vi "Setup manipulator (SubVI).vi"(1 "G_upper bound":i32, 3 "M_lower bound":i32, 11 "error in (no error)":errorcluster, 12 "M_Encoder Ref In":T1, 14 "G_Encoder Ref In":T1) -> (15 "error out":errorcluster)   [LabVIEW 2017]
uses:
  <vilib>/myRIO/Instrument Drivers/Onboard IO/Encoder/typedefs/Encoder Reference.ctl
  <vilib>/myRIO/Common/Instrument Driver Framework/Utilities/typedefs/myRIO Generic Hardware Reference.ctl
  <vilib>/myRIO/Common/Instrument Driver Framework/Utilities/typedefs/Hardware Version Enum.ctl
  <vilib>/myRIO/Common/Instrument Driver Framework/Utilities/typedefs/myRIO v1.0 Reference.ctl
  <vilib>/myRIO/Common/Instrument Driver Framework/Utilities/typedefs/Generic FPGA Reference.ctl
  <vilib>/myRIO/Common/Instrument Driver Framework/myRIO v1.0/Encoder/typedefs/Encoder Channels Enum.ctl
  <vilib>/myRIO/Instrument Drivers/Onboard IO/DIO/typedefs/DIO Reference.ctl
  <vilib>/myRIO/Common/Instrument Driver Framework/myRIO v1.0/DIO/typedefs/DIO Channels List.ctl
  <vilib>/myRIO/Common/Instrument Driver Framework/myRIO v1.0/DIO/typedefs/DIO Channels Enum.ctl
  <vilib>/userdefined/High Color/nirio_resource_hc.ctl
  <vilib>/myRIO/Common/Instrument Driver Framework/Utilities/vis/Is FPGA Ref Available.vi
  <vilib>/myRIO/Common/Instrument Driver Framework/myRIO v1.0/DIO/vis/myRIO v1.1 Open DIO.vi
  <vilib>/myRIO/Instrument Drivers/Onboard IO/DIO/vis/Write.vi
  <vilib>/myRIO/Common/Instrument Driver Framework/Utilities/vis/Validate Channels.vi
  <vilib>/myRIO/Common/Instrument Driver Framework/myRIO v1.0/DIO/vis/myRIO v1.0 Reserve DIO.vi
  <vilib>/myRIO/Common/Instrument Driver Framework/myRIO v1.0/Resource Manager/vis/myRIO v1.0 Reserve Channel List.vi
  <vilib>/myRIO/Common/Instrument Driver Framework/myRIO v1.0/DIO/vis/myRIO v1.0 Build MUX Configuration DIO.vi
  <vilib>/myRIO/Common/Instrument Driver Framework/myRIO v1.0/Resource Manager/vis/myRIO v1.0 Reserve Channel.vi
  <vilib>/myRIO/Common/Instrument Driver Framework/myRIO v1.0/Resource Manager/vis/myRIO v1.0 Unreserve Channel.vi
  <vilib>/myRIO/Common/Instrument Driver Framework/myRIO v1.0/Resource Manager/vis/myRIO v1.0 Create Configuration List.vi
  <vilib>/myRIO/Common/Instrument Driver Framework/myRIO v1.0/Resource Manager/vis/myRIO v1.0 Build Mutex Name.vi
  <vilib>/Utility/error.llb/Error Cluster From Error Code.vi
  <vilib>/myRIO/Common/Instrument Driver Framework/myRIO v1.0/Encoder/vis/myRIO v1.0 Read Encoder.vi
  <vilib>/Utility/VariantDataType/GetNumericInfo.vi
  <vilib>/myRIO/Common/Instrument Driver Framework/myRIO v1.0/myRIO v1.1 Open.vi
  <vilib>/myRIO/Common/Instrument Driver Framework/Utilities/vis/IO Manager.vi
  <vilib>/myRIO/Common/Instrument Driver Framework/Utilities/vis/Configuration Manager.vi
  <vilib>/myRIO/Common/Instrument Driver Framework/myRIO v1.0/Resource Manager/vis/myRIO v1.0 Configure IO.vi
  <vilib>/myRIO/Common/Instrument Driver Framework/myRIO v1.0/myRIO v1.0 Close.vi
  <vilib>/myRIO/Common/Instrument Driver Framework/myRIO v1.0/DIO/vis/myRIO v1.0 Write DIO.vi
  <vilib>/myRIO/Express VI/Onboard IO/DO/DO Express VI.xnode
  <vilib>/myRIO/Instrument Drivers/Onboard IO/DIO/vis/myRIO DIO Open.xnode
  <vilib>/myRIO/Instrument Drivers/Onboard IO/Encoder/Encoder.lvlib
  <vilib>/myRIO/Instrument Drivers/Onboard IO/DIO/DIO.lvlib
panel:
  out "reversedG":bool
  out "reversedM":bool
  in  "offset for Extra Stop":i32=100
  in  "iterations control":i32=10
  in  "offset":i32=50
  in  "frames to pass":i32=100
  in  "def it":i32=100
  out "ArrG_enc_val":i32[](array[numeric])
  out "ArrM_enc_val":i32[](array[numeric])
  in  "G+ (B/DIO13 (Pin 26))":bool
  in  "G- (B/DIO7 (Pin 25))":bool
  in  "M- (B/DIO6 (Pin 23))":bool
  in  "M+ (B/DIO5 (Pin 21))":bool
  in  "stopG":bool
  out "G+":bool
  out "G enc val":i32
  out "M+":bool
  in  "stopM":bool
  out "M enc val":i32
  # "EXTRA STOP CONTROLS"
  # "SET UP THE VALUES"
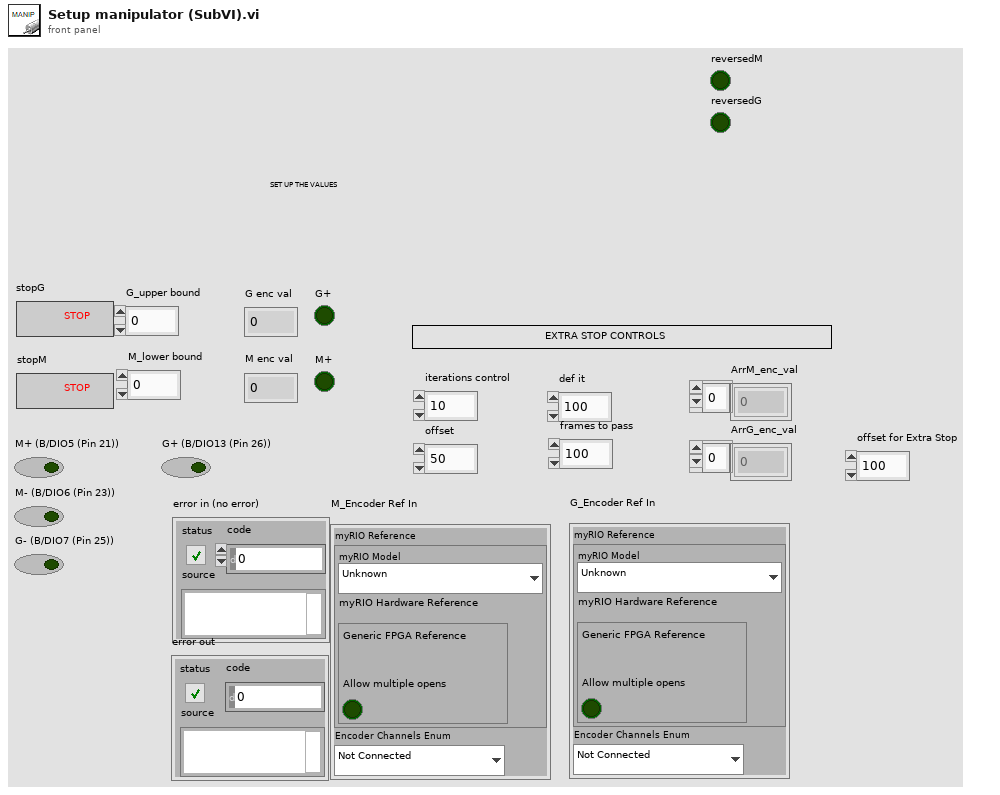
[diagram p1: front panel]
types:
  T1 = typedef "Encoder.lvlib/Encoder Reference.ctl" = cluster{"myRIO Reference":T2, "Encoder Channels Enum":T6}
  T2 = typedef "myRIO Generic Hardware Reference.ctl" = cluster{"myRIO Model":T3, "myRIO Hardware Reference":T4}
  T3 = typedef "Hardware Version Enum.ctl" = enum16{"Unknown", "myRIO-1900", "myRIO-1950", "roboRIO", "NI ELVIS RIO CM"}
  T4 = typedef "myRIO v1.0 Reference.ctl" = cluster{"Generic FPGA Reference":T5, "Allow multiple opens":bool}
  T5 = typedef "Generic FPGA Reference.ctl" = refnum<k20>
  T6 = typedef "Encoder Channels Enum.ctl" = enum16{"Not Connected", "C/ENC0", "C/ENC1", "A/ENC", "B/ENC", "DIO/ENC0", "DIO/ENC1", "DIO/ENC2", "DIO/ENC3", "DIO/ENC4"}
  T7 = typedef "DIO.lvlib/DIO Reference.ctl" = cluster{"myRIO Reference":T2, "DIO Channels List":T8}
  T8 = typedef "DIO Channels List.ctl" = T9[]
  T9 = typedef "DIO Channels Enum.ctl" = enum16{"Not Connected", "C/DIO0", "C/DIO1", "C/DIO2", "C/DIO3", "C/DIO4", "C/DIO5", "C/DIO6", "C/DIO7", "A/DIO0", "A/DIO1", "A/DIO2", "A/DIO3", "A/DIO4", "A/DIO5", "A/DIO6", "A/DIO7", "A/DIO8", "A/DIO9", "A/DIO10", "A/DIO11", "A/DIO12", "A/DIO13", "A/DIO14", "A/DIO15", "B/DIO0", "B/DIO1", "B/DIO2", "B/DIO3", "B/DIO4", "B/DIO5", "B/DIO6", "B/DIO7", "B/DIO8", "B/DIO9", "B/DIO10", "B/DIO11", "B/DIO12", "B/DIO13", "B/DIO14", "B/DIO15", "LED0", "LED1", "LED2", "LED3", "Button0", "DIO/DIO0", "DIO/DIO1", "DIO/DIO2", "DIO/DIO3", "DIO/DIO4", "DIO/DIO5", "DIO/DIO6", "DIO/DIO7", "DIO/DIO8", "DIO/DIO9", "SPI/CS0", "SPI/CS1", "SPI/CS2", "SPI/CS3", "LED RADIO (Green)", "LED RADIO (Red)", "LED COMM (Green)", "LED COMM (Red)", "LED MODE (Green)", "LED MODE (Red)"}
  T10 = typedef "nirio_resource_hc.ctl" = tag
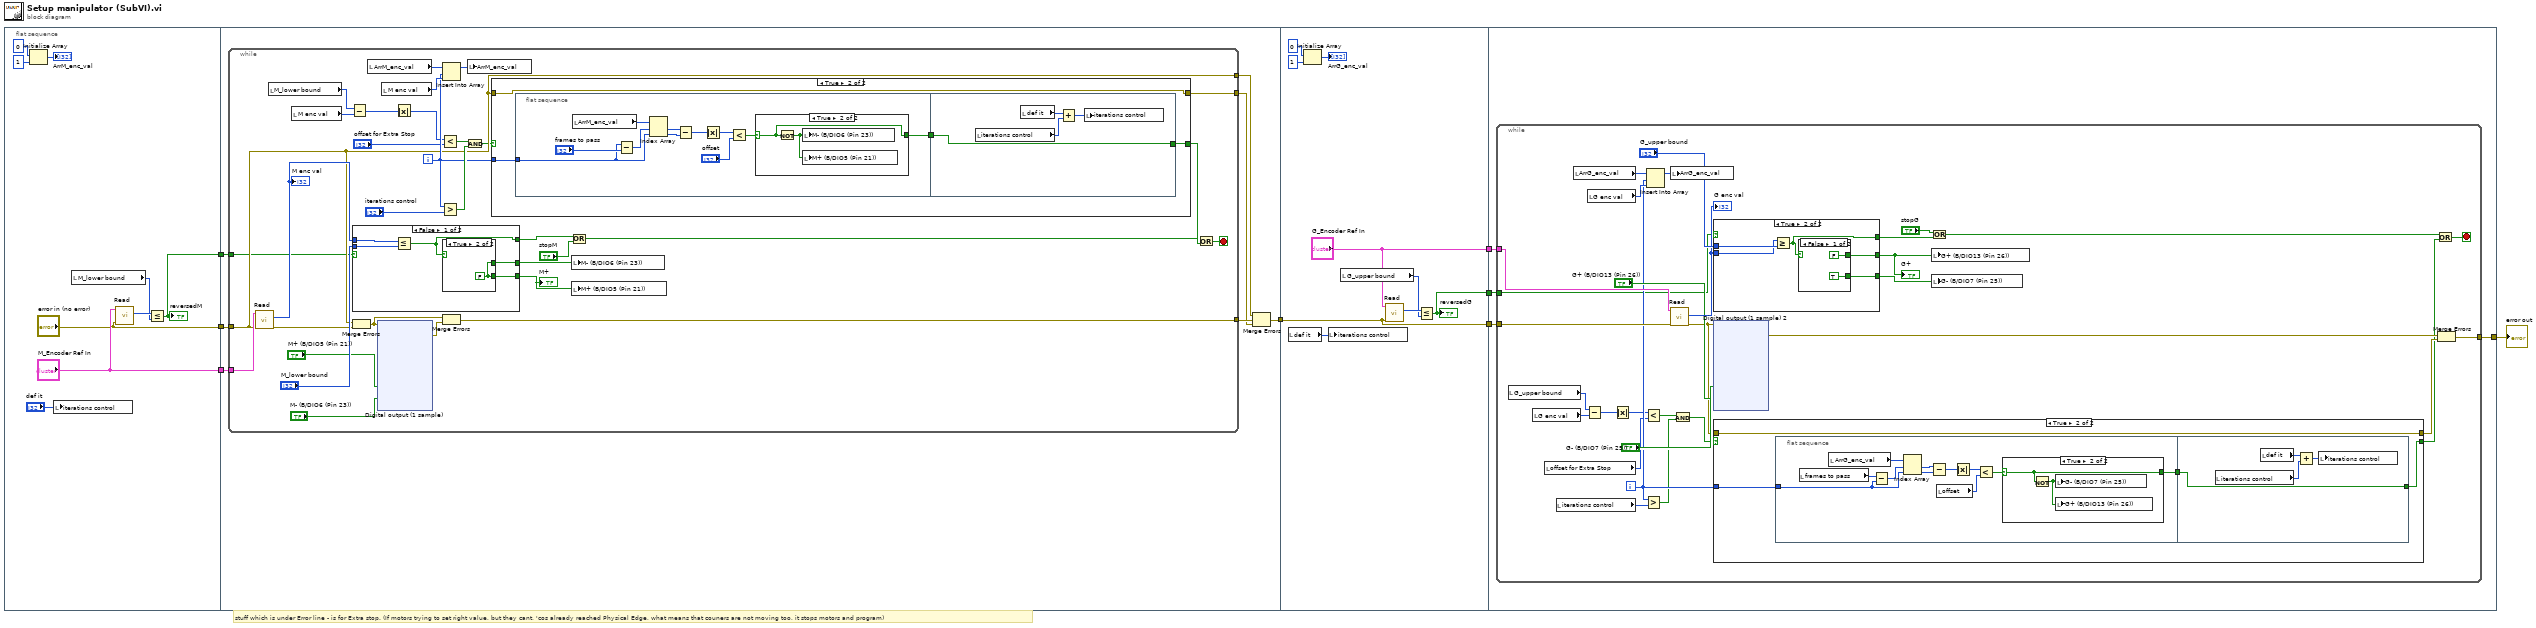
[diagram p0: block diagram]
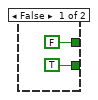
[diagram p4: hidden frame]
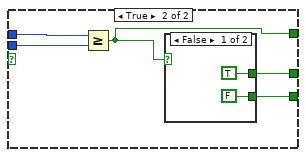
[diagram p5: hidden frame]
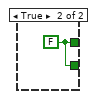
[diagram p6: hidden frame]
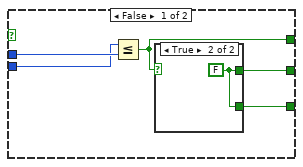
[diagram p9: hidden frame]
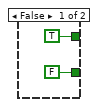
[diagram p10: hidden frame]
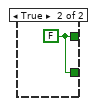
[diagram p11: hidden frame]
diagram:
  # "stuff which is under Error line - is for Extra stop. (If motors trying to set right value, but they cant, 'cos already reached Physical Edge, what means that couners are not moving too, it stops motors and program)"
  n1 = flat-sequence {
    tunnel: ["error in (no error)"] -> w8
    tunnel: ["M_Encoder Ref In"] -> w7
    tunnel: [w9] -> w1
    tunnel: w8 -> [w24]
    tunnel: w7 -> [w21]
    tunnel: [w20] -> w6
    tunnel: w1 -> [w18]
    tunnel: w6 -> [w136]
    tunnel: [w136] -> w5
    tunnel: ["G_Encoder Ref In"] -> w4
    tunnel: [w133] -> w2
    tunnel: w5 -> [w145]
    tunnel: w4 -> [w144]
    tunnel: [w143] -> w3
    tunnel: w2 -> [w142]
    frame #0 {
      n2 = Initialize Array(0 ("dimension size"), 1 ("dimension size")) -> (→"ArrM_enc_val":i32[])
      n3 = local write "iterations control"("def it") -> ()
      n4 = local read "M_lower bound"() -> (w10:i32)
      n5 = call <vilib>:"Read.vi"("error in (no error)"="error in (no error)", "Encoder Ref In"="M_Encoder Ref In") -> ("Counter Value"=w11:i32)  [unwired: 5 in, 4 out]
      n6 = Less Or Equal?(x=w11, y=w10) -> (x <= y?=w9:bool)
      "reversedM" <- w9
    }
    frame #1 {
      n7 = while {
        tunnel: w24 -> [w40]
        tunnel: [w40] -> w23
        tunnel: [w55] -> w22
        tunnel: w21 -> [w54]
        tunnel: [w39] -> w19
        tunnel: w18 -> [w25]
        i -> [w41]
        stop <- w37 stop-if-true
        n8 = call <vilib>:"Read.vi"("error in (no error)"=w40, "Encoder Ref In"=w54) -> ("error out"=w53:errorcluster, "Counter Value"=w52:i32)  [unwired: 5 in, 3 out]
        "M enc val" <- w52
        n9 = local read "M_lower bound"() -> (w30:i32)
        n10 = local read "M enc val"() -> (w31:i32)
        n11 = Subtract(x=w30, y=w31) -> (x-y=w28:i32)
        n12 = case shown="False" w25 {
          tunnel: "M_lower bound" -> [w85 w93]
          tunnel: [w81 w89] -> w48
          tunnel: w52 -> [w84 w92]
          tunnel: [w83 w90] -> w34
          tunnel: [w82 w91] -> w33
          frame False {
            n13 = Less Or Equal?(x=w84, y=w85) -> (x <= y?=w81:bool)
            n14 = case shown="True" w81 {
              tunnel: [TRUE w88] -> w83
              tunnel: [FALSE w88] -> w82
              frame False {
              }
              frame True {
                w88 = FALSE
              }
            }
          }
          frame True {
            n15 = Greater Or Equal?(x=w92, y=w93) -> (x >= y?=w89:bool)
            n16 = case shown="False" w89 {
              tunnel: [TRUE ("M- (B/DIO6 (Pin 23))") w96] -> w91
              tunnel: [FALSE ("M- (B/DIO6 (Pin 23))") w96] -> w90
              frame False {
              }
              frame True {
                w96 = FALSE
              }
            }
          }
        }
        "M+" <- w34
        n17 = Merge Errors(w40, w53) -> (w49:errorcluster)
        n18 = local read "ArrM_enc_val"() -> (w44:i32[])
        n19 = xnode "Digital output (1 sample)"("M+ (B/DIO5 (Pin 21))"="M+ (B/DIO5 (Pin 21))", "M- (B/DIO6 (Pin 23))"="M- (B/DIO6 (Pin 23))", "error in (no error)"=w49) -> ("error out"=w50:errorcluster)
        n20 = local read "M enc val"() -> (w42:i32)
        n21 = Absolute Value(x=w28) -> (abs(x)=w26:i32)
        n22 = Less?(x=w26, y="offset for Extra Stop") -> (x < y?=w29:bool)
        n23 = Greater?(x=w41, y="iterations control") -> (0:w46:bool)
        n24 = Insert Into Array(array=w44, index=w41, new element=w42) -> (w43:i32[])
        n25 = Merge Errors(w49, w50) -> (w55:errorcluster)
        n26 = And(x=w29, y=w46) -> (x .and. y?=w32:bool)
        n27 = local write "ArrM_enc_val"(w43) -> ()
        n28 = case shown="True" w32 {
          selector: w32 -> [w57 _]
          tunnel: w41 -> [_ w62]
          tunnel: w40 -> [w58 w61]
          tunnel: [w58 w61] -> w39
          tunnel: [w57 w59] -> w47
          frame False {
          }
          frame True {
            n29 = flat-sequence {
              tunnel: w62 -> [w70]
              tunnel: [w63] -> w60
              tunnel: [w77] -> w59
              tunnel: w60 -> [w77]
              frame #0 {
                n30 = local read "ArrM_enc_val"() -> (w73:i32[])
                n31 = Subtract(x=w70, y="frames to pass") -> (x-y=w71:i32)
                n32 = Index Array(array=w73, index #1=w71, index #2=w70) -> (element #1=w69:i32, element #2=w68:i32)
                n33 = Subtract(x=w69, y=w68) -> (x-y=w67:i32)
                n34 = Absolute Value(x=w67) -> (abs(x)=w66:i32)
                n35 = Less?(x=w66, y="offset") -> (x < y?=w64:bool)
                n36 = case shown="True" w64 {
                  selector: w64 -> [w74 w75]
                  tunnel: [w74 w75] -> w63
                  frame False {
                  }
                  frame True {
                    n37 = Not(x=w75) -> (.not. x?=w76:bool)
                    n38 = local write "M- (B/DIO6 (Pin 23))"(w76) -> ()
                    n39 = local write "M+ (B/DIO5 (Pin 21))"(w76) -> ()
                  }
                }
              }
              frame #1 {
                n40 = local read "iterations control"() -> (w80:i32)
                n41 = local read "def it"() -> (w78:i32)
                n42 = Add(x=w78, y=w80) -> (x+y=w79:i32)
                n43 = local write "iterations control"(w79) -> ()
              }
            }
          }
        }
        n44 = Or(x=w48, y="stopM") -> (x .or. y?=w38:bool)
        n45 = local write "M- (B/DIO6 (Pin 23))"(w33) -> ()
        n46 = local write "M+ (B/DIO5 (Pin 21))"(w34) -> ()
        n47 = Or(x=w38, y=w47) -> (x .or. y?=w37:bool)
      }
      n48 = Merge Errors(w23, w22, w19) -> (w20:errorcluster)
    }
    frame #2 {
      n49 = local read "def it"() -> (w139:i32)
      n50 = Initialize Array(0 ("dimension size"), 1 ("dimension size")) -> (→"ArrG_enc_val":i32[])
      n51 = local write "iterations control"(w139) -> ()
      n52 = local read "G_upper bound"() -> (w134:i32)
      n53 = call <vilib>:"Read.vi"("error in (no error)"=w136, "Encoder Ref In"="G_Encoder Ref In") -> ("Counter Value"=w135:i32)  [unwired: 5 in, 4 out]
      n54 = Less Or Equal?(x=w135, y=w134) -> (x <= y?=w133:bool)
      "reversedG" <- w133
    }
    frame #3 {
      n55 = while {
        tunnel: w145 -> [w174]
        tunnel: [w159] -> w143
        tunnel: w144 -> [w170]
        tunnel: w142 -> [w146]
        i -> [w161]
        stop <- w156 stop-if-true
        n56 = local read "G_upper bound"() -> (w150:i32)
        n57 = local read "G enc val"() -> (w151:i32)
        n58 = local read "offset for Extra Stop"() -> (w149:i32)
        n59 = local read "iterations control"() -> (w163:i32)
        n60 = local read "ArrG_enc_val"() -> (w164:i32[])
        n61 = Subtract(x=w150, y=w151) -> (x-y=w152:i32)
        n62 = local read "G enc val"() -> (w165:i32)
        n63 = Absolute Value(x=w152) -> (abs(x)=w147:i32)
        n64 = Less?(x=w147, y=w149) -> (x < y?=w148:bool)
        n65 = Greater?(x=w161, y=w163) -> (0:w157:bool)
        n66 = Insert Into Array(array=w164, index=w161, new element=w165) -> (w162:i32[])
        n67 = local write "ArrG_enc_val"(w162) -> ()
        n68 = call <vilib>:"Read.vi"("error in (no error)"=w174, "Encoder Ref In"=w170) -> ("error out"=w160:errorcluster, "Counter Value"=w175:i32)  [unwired: 5 in, 3 out]
        "G enc val" <- w175
        n69 = And(x=w148, y=w157) -> (x .and. y?=w153:bool)
        n70 = case shown="True" w146 {
          tunnel: "G_upper bound" -> [w205 w213]
          tunnel: w175 -> [w204 w212]
          tunnel: [w201 w209] -> w172
          tunnel: [w203 w210] -> w167
          tunnel: [w202 w211] -> w166
          frame False {
            n71 = Less Or Equal?(x=w204, y=w205) -> (x <= y?=w201:bool)
            n72 = case shown="True" w201 {
              tunnel: [TRUE w208] -> w203
              tunnel: [FALSE w208] -> w202
              frame False {
              }
              frame True {
                w208 = FALSE
              }
            }
          }
          frame True {
            n73 = Greater Or Equal?(x=w212, y=w213) -> (x >= y?=w209:bool)
            n74 = case shown="False" w209 {
              tunnel: [TRUE w216] -> w211
              tunnel: [FALSE w216] -> w210
              frame False {
              }
              frame True {
                w216 = FALSE
              }
            }
          }
        }
        "G+" <- w167
        n75 = xnode "Digital output (1 sample) 2"("G- (B/DIO7 (Pin 25))"="G- (B/DIO7 (Pin 25))", "G+ (B/DIO13 (Pin 26))"="G+ (B/DIO13 (Pin 26))", "error in (no error)"=w160) -> ("error out"=w171:errorcluster)
        n76 = case shown="True" w153 {
          selector: w153 -> [w177 _]
          tunnel: w161 -> [_ w182]
          tunnel: w160 -> [w178 w181]
          tunnel: [w178 w181] -> w158
          tunnel: [w177 w180] -> w154
          frame False {
          }
          frame True {
            n77 = flat-sequence {
              tunnel: w182 -> [w188]
              tunnel: [w183] -> w179
              tunnel: [w197] -> w180
              tunnel: w179 -> [w197]
              frame #0 {
                n78 = local read "frames to pass"() -> (w186:i32)
                n79 = local read "ArrG_enc_val"() -> (w193:i32[])
                n80 = Subtract(x=w186, y=w188) -> (x-y=w187:i32)
                n81 = Index Array(array=w193, index #1=w187, index #2=w188) -> (element #1=w190:i32, element #2=w185:i32)
                n82 = Subtract(x=w190, y=w185) -> (x-y=w192:i32)
                n83 = local read "offset"() -> (w184:i32)
                n84 = Absolute Value(x=w192) -> (abs(x)=w191:i32)
                n85 = Less?(x=w191, y=w184) -> (x < y?=w189:bool)
                n86 = case shown="True" w189 {
                  selector: w189 -> [w194 w195]
                  tunnel: [w194 w195] -> w183
                  frame False {
                  }
                  frame True {
                    n87 = Not(x=w195) -> (.not. x?=w196:bool)
                    n88 = local write "G- (B/DIO7 (Pin 25))"(w196) -> ()
                    n89 = local write "G+ (B/DIO13 (Pin 26))"(w196) -> ()
                  }
                }
              }
              frame #1 {
                n90 = local read "iterations control"() -> (w199:i32)
                n91 = local read "def it"() -> (w198:i32)
                n92 = Add(x=w198, y=w199) -> (x+y=w200:i32)
                n93 = local write "iterations control"(w200) -> ()
              }
            }
          }
        }
        n94 = Or(x="stopG", y=w172) -> (x .or. y?=w155:bool)
        n95 = local write "G+ (B/DIO13 (Pin 26))"(w167) -> ()
        n96 = local write "G- (B/DIO7 (Pin 25))"(w166) -> ()
        n97 = Or(x=w155, y=w154) -> (x .or. y?=w156:bool)
        n98 = Merge Errors(w171, w158) -> (w159:errorcluster)
      }
    }
  }
  "error out" <- w3
